vi "json Insert String Array - array path.vi"(8 "error in (no error)":errorcluster, 9 "anything":string[](array[string]), 10 "path":string[](array[string]), 11 "JSON Document in":refnum<class "JSON Document.lvclass">) -> (0 "error out":errorcluster, 1 "replaced?":bool, 3 "JSON Document out":refnum<class "JSON Document.lvclass">)   [LabVIEW 2015, in "JSON Document.lvclass"]
uses:
  JSON Document.lvclass
  json Insert String Array - string path.vi
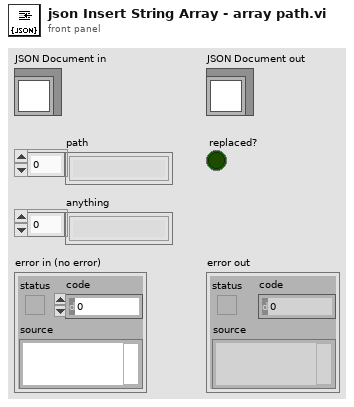
[diagram p1: front panel]
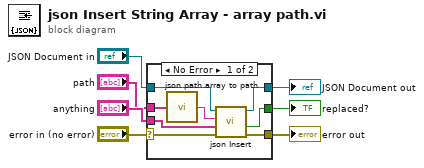
[diagram p0: block diagram]
diagram:
  n1 = case shown="No Error" "error in (no error)" {
    selector: "error in (no error)" -> [w11 w17]
    tunnel: [w12 w17] -> w6
    tunnel: [w14 w16] -> w4
    tunnel: "JSON Document in" -> [w15 w16]
    tunnel: "anything" -> [w10 _]
    tunnel: "path" -> [w9 _]
    tunnel: [w13 _] -> w1
    frame No Error {
      n2 = call "json path array to path.vi"("path"=w9) -> ("String"=w8:string)
      n3 = call-poly "json Insert.vi"("error in (no error)"=w11, "anything"=w10, "path"=w8, "JSON Document in"=w15) -> ("error out"=w12:errorcluster, "replaced?"=w13:bool, "JSON Document out"=w14:refnum<class "JSON Document.lvclass">)  [unwired: 5 in]
    }
    frame Error {
    }
  }
  "error out" <- w6
  "JSON Document out" <- w4
  "replaced?" <- w1
